vi "Lector_Ingen.vi"() -> ()   [LabVIEW 2017, in "Lib_Maestro_Ingen.lvlib"]
uses:
  Lib_Maestro_Ingen.lvlib
panel:
  in  "000001":bool
  in  "400001":u16
  in  "Tab Control 3":enum32{"Registro", "Control de variables"}(tab)=enum."Control de variables"
  in  "Tab Control":T1(tab)=enum."Registro de Frecuencia"
  out "Voltaje Fase 3":dbl(graph)=119.45
  out "Voltaje Fase 2":dbl(graph)=135.24
  out "Voltaje Fase 1":dbl(graph)=134.03
  out "Voltaje Promedio":dbl(graph)=233.23
  out "Corriente Promedio":dbl(graph)=53.75
  out "Corriente Fase 1":dbl(graph)=60.84
  out "Corriente Fase 2":dbl(graph)=61.24
  out "Corriente Fase 3":dbl(graph)=39.16
  out "Potencia Fase 3":dbl(graph)=76.8
  out "Potencia Fase 2":dbl(graph)=84.51
  out "Potencia Fase 1":dbl(graph)=83.64
  out "Potencia Promedio":dbl(graph)=81.65
  out "Factor de Potencia Fase 3":dbl(graph)=90.57
  out "Factor de Potencia Fase 2":dbl(graph)=90.84
  out "Factor de Potencia Fase 1":dbl(graph)=90.36
  out "Factor de Potencia Promedio":dbl(graph)=90.59
  out "Frecuencia":dbl(graph)=60.18
  in  "Tab Control 2":T2(tab)
  in  "CONTROL TEMPERATURA":cluster{"SET POINT":dbl, "INC T":dbl}={"SET POINT"=50.0, "INC T"=1.0}
  out "TEMPERATURA ACTUAL":dbl(slide)=31.0 scale=0.0..100.0
  out "Tempratura":cluster{"Dato":dbl, "SET POINT":dbl}(graph)
  out "Presion":cluster{"Dato":dbl, "SET POINT":dbl}(graph)
  in  "CONTROL DE PRESIÓN":cluster{"SET POINT":dbl, "INC P":dbl}={"SET POINT"=50.0, "INC P"=1.0}
  out "PRESIÓN ACTUAL":dbl(knob)=50.0 scale=0.0..200.0
  out "Humedad":cluster{"Dato":dbl, "SET POINT":dbl}(graph)
  in  "CONTROL DE HUMEDAD":cluster{"SET POINT":dbl, "INC %":dbl}={"SET POINT"=50.0, "INC %"=1.0}
  out "HUMEDAD ACTUAL":dbl(knob)=50.0 scale=0.0..100.0
  out "Volumen":cluster{"Dato":dbl, "SET POINT":dbl}(graph)
  in  "CONTROL DE LLENADO":cluster{"SET POINT":dbl, "INC  L":dbl}={"SET POINT"=25.0, "INC  L"=1.0}
  out "VOLUMEN ACTUAL":dbl(slide)=25.0 scale=0.0..100.0
  in  "Stop":bool
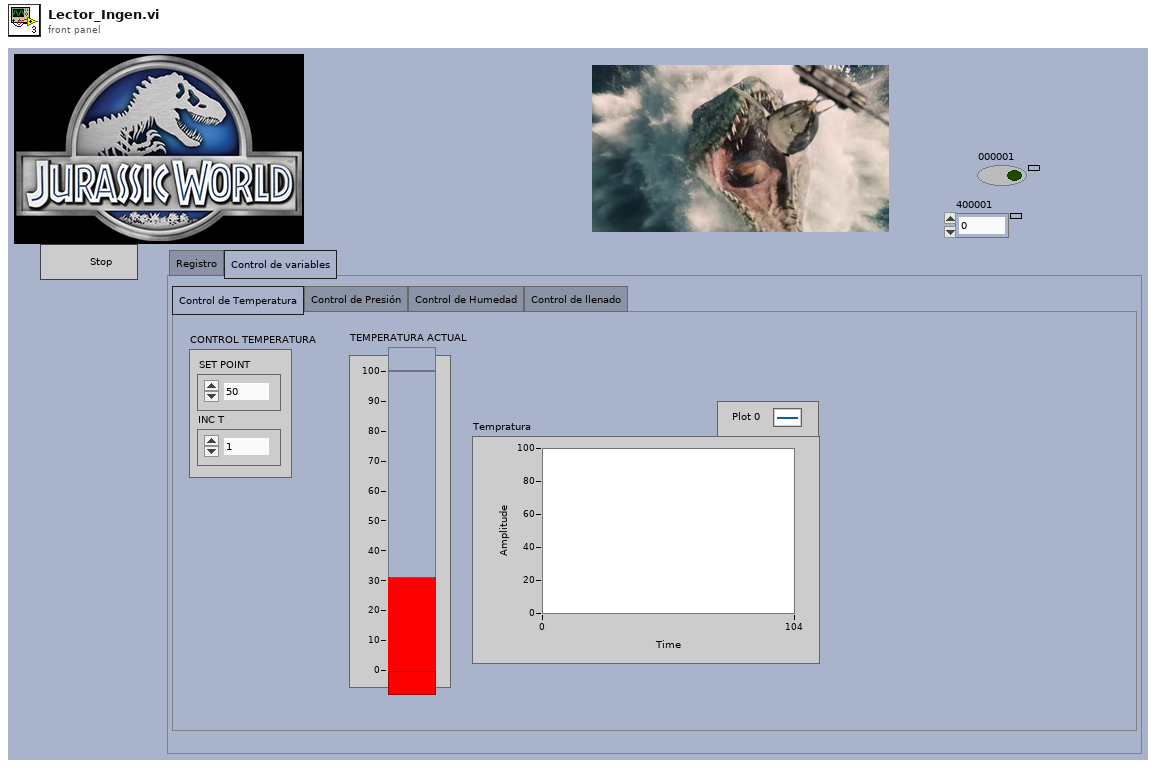
[diagram p1: front panel]
types:
  T1 = enum32{"Registro de Tensión", "Registro de Corriente", "Registro de Potencia", "Registro de Factor de Potencia", "Registro de Frecuencia"}
  T2 = enum32{"Control de Temperatura", "Control de Presión", "Control de Humedad", "Control de llenado"}
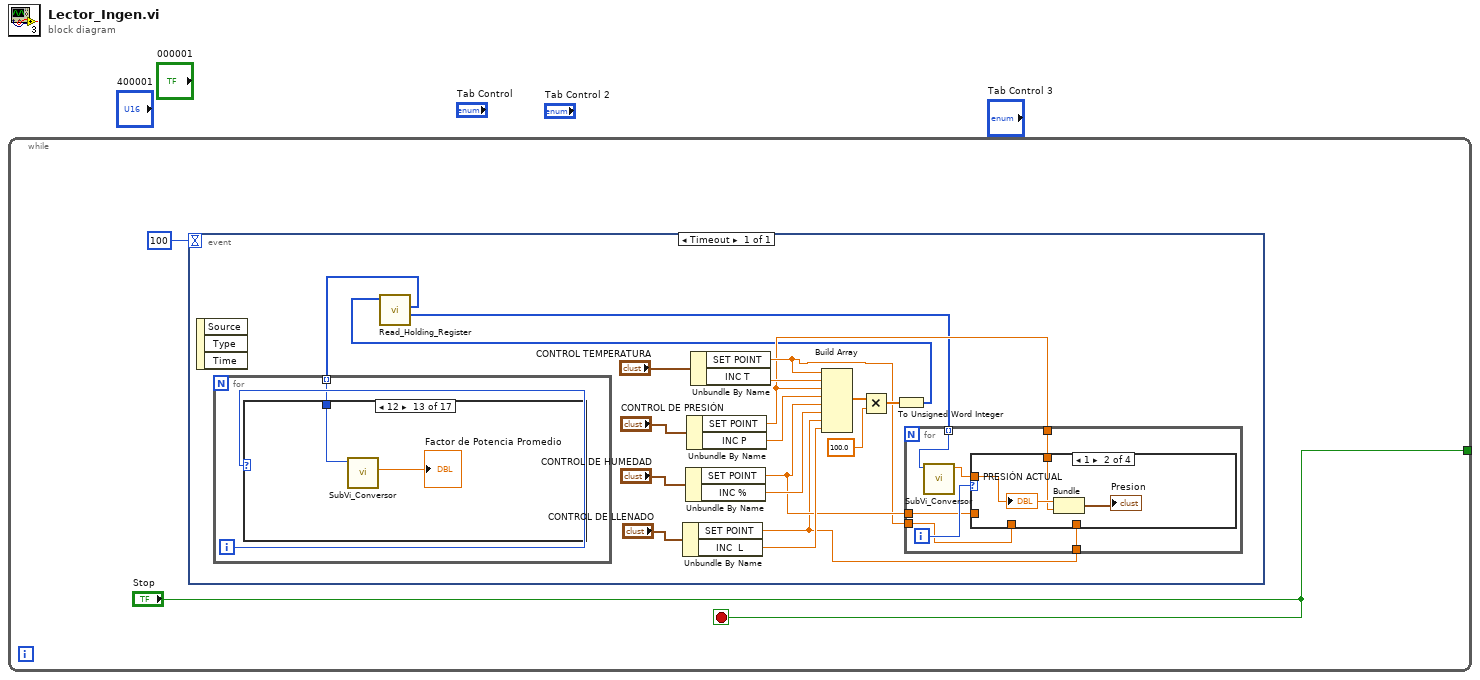
[diagram p0: block diagram]
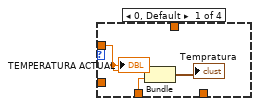
[diagram p2: hidden frame]
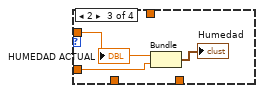
[diagram p3: hidden frame]
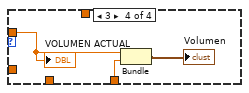
[diagram p4: hidden frame]
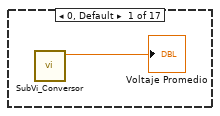
[diagram p5: hidden frame]
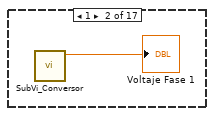
[diagram p6: hidden frame]
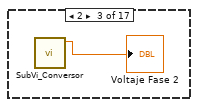
[diagram p7: hidden frame]
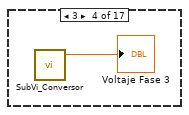
[diagram p8: hidden frame]
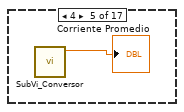
[diagram p9: hidden frame]
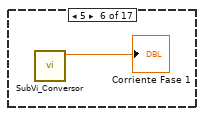
[diagram p10: hidden frame]
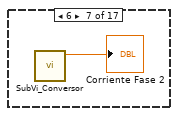
[diagram p11: hidden frame]
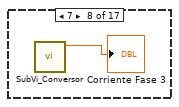
[diagram p12: hidden frame]
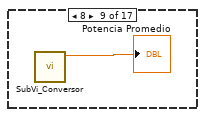
[diagram p13: hidden frame]
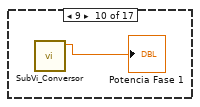
[diagram p14: hidden frame]
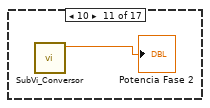
[diagram p15: hidden frame]
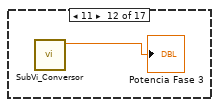
[diagram p16: hidden frame]
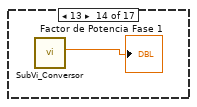
[diagram p17: hidden frame]
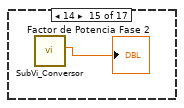
[diagram p18: hidden frame]
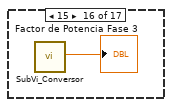
[diagram p19: hidden frame]
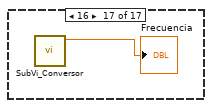
[diagram p20: hidden frame]
diagram:
  n1 = while {
    tunnel: ["Stop"] -> _
    stop <- "Stop" stop-if-true
    n2 = event shown="[0] Timeout" {
      selector: _ -> [_]
      dyn-events: _ -> [_]
      timeout: 100 -> [_]
      event Timeout {
        n3 = event-data() -> ()  [unwired: 1 in, 3 out]
        n4 = Unbundle By Name("CONTROL DE LLENADO") -> ("SET POINT"=w8:dbl, "INC  L"=w13:dbl)
        n5 = Unbundle By Name("CONTROL DE HUMEDAD") -> ("SET POINT"=w9:dbl, "INC %"=w14:dbl)
        n6 = Unbundle By Name("CONTROL DE PRESIÓN") -> ("SET POINT"=w6:dbl, "INC P"=w15:dbl)
        n7 = Unbundle By Name("CONTROL TEMPERATURA") -> ("SET POINT"=w7:dbl, "INC T"=w16:dbl)
        n8 = Build Array(w7, w16, w6, w15, w9, w14, w8, w13) -> (w12:dbl[])
        n9 = Multiply(x=w12, y=100.0) -> (x*y=w10:dbl[])
        n10 = To Unsigned Word Integer(number=w10) -> (unsigned 16bit integer=w5:u16[])
        n11 = call "Read_Holding_Register.vi"("Escritura_Variables"=w5) -> ("Registros_B"=w3:u16[], "Registros_A"=w4:u16[])  [unwired: 7 in, 1 out]
        n12 = for {
          tunnel: w4 -> [w40] mode=indexing
          i -> [w41]
          n13 = case shown="12" w41 {
            tunnel: w40 -> [_ _ _ _ _ _ _ _ _ _ _ _ w54 _ _ _ _]
            frame 0, Default {
              n14 = call "SubVi_Conversor.vi"() -> ("Dato"=→"Voltaje Promedio":dbl)  [unwired: 10 in, 1 out]
            }
            frame 1 {
              n15 = call "SubVi_Conversor.vi"() -> ("Dato"=→"Voltaje Fase 1":dbl)  [unwired: 10 in, 1 out]
            }
            frame 2 {
              n16 = call "SubVi_Conversor.vi"() -> ("Dato"=→"Voltaje Fase 2":dbl)  [unwired: 10 in, 1 out]
            }
            frame 3 {
              n17 = call "SubVi_Conversor.vi"() -> ("Dato"=→"Voltaje Fase 3":dbl)  [unwired: 10 in, 1 out]
            }
            frame 4 {
              n18 = call "SubVi_Conversor.vi"() -> ("Dato"=→"Corriente Promedio":dbl)  [unwired: 10 in, 1 out]
            }
            frame 5 {
              n19 = call "SubVi_Conversor.vi"() -> ("Dato"=→"Corriente Fase 1":dbl)  [unwired: 10 in, 1 out]
            }
            frame 6 {
              n20 = call "SubVi_Conversor.vi"() -> ("Dato"=→"Corriente Fase 2":dbl)  [unwired: 10 in, 1 out]
            }
            frame 7 {
              n21 = call "SubVi_Conversor.vi"() -> ("Dato"=→"Corriente Fase 3":dbl)  [unwired: 10 in, 1 out]
            }
            frame 8 {
              n22 = call "SubVi_Conversor.vi"() -> ("Dato"=→"Potencia Promedio":dbl)  [unwired: 10 in, 1 out]
            }
            frame 9 {
              n23 = call "SubVi_Conversor.vi"() -> ("Dato"=→"Potencia Fase 1":dbl)  [unwired: 10 in, 1 out]
            }
            frame 10 {
              n24 = call "SubVi_Conversor.vi"() -> ("Dato"=→"Potencia Fase 2":dbl)  [unwired: 10 in, 1 out]
            }
            frame 11 {
              n25 = call "SubVi_Conversor.vi"() -> ("Dato"=→"Potencia Fase 3":dbl)  [unwired: 10 in, 1 out]
            }
            frame 12 {
              n26 = call "SubVi_Conversor.vi"("Entrada_U16"=w54) -> ("Factor_de_potencia"=→"Factor de Potencia Promedio":dbl)  [unwired: 9 in, 1 out]
            }
            frame 13 {
              n27 = call "SubVi_Conversor.vi"() -> ("Factor_de_potencia"=→"Factor de Potencia Fase 1":dbl)  [unwired: 10 in, 1 out]
            }
            frame 14 {
              n28 = call "SubVi_Conversor.vi"() -> ("Factor_de_potencia"=→"Factor de Potencia Fase 2":dbl)  [unwired: 10 in, 1 out]
            }
            frame 15 {
              n29 = call "SubVi_Conversor.vi"() -> ("Factor_de_potencia"=→"Factor de Potencia Fase 3":dbl)  [unwired: 10 in, 1 out]
            }
            frame 16 {
              n30 = call "SubVi_Conversor.vi"() -> ("Dato"=→"Frecuencia":dbl)  [unwired: 10 in, 1 out]
            }
          }
        }
        n31 = for {
          tunnel: w9 -> [w25]
          tunnel: w8 -> [w24]
          tunnel: w7 -> [w23]
          tunnel: w6 -> [w22]
          tunnel: w3 -> [w21] mode=indexing
          i -> [w27]
          n32 = call "SubVi_Conversor.vi"("Entrada_U16"=w21) -> ("Dato"=w26:dbl)  [unwired: 9 in, 1 out]
          n33 = case shown="1" w27 {
            tunnel: w26 -> [w29 w32 w36 w38]
            tunnel: w25 -> [_ _ w34 _]
            tunnel: w24 -> [_ _ _ w37]
            tunnel: w23 -> [w28 _ _ _]
            tunnel: w22 -> [_ w31 _ _]
            frame 0, Default {
              n34 = Bundle("Dato"=w29, "SET POINT"=w28) -> (→"Tempratura":cluster{"Dato":dbl, "SET POINT":dbl})  [unwired: 1 in]
              "TEMPERATURA ACTUAL" <- w29
            }
            frame 1 {
              n35 = Bundle("Dato"=w32, "SET POINT"=w31) -> (→"Presion":cluster{"Dato":dbl, "SET POINT":dbl})  [unwired: 1 in]
              "PRESIÓN ACTUAL" <- w32
            }
            frame 2 {
              n36 = Bundle("Dato"=w36, "SET POINT"=w34) -> (→"Humedad":cluster{"Dato":dbl, "SET POINT":dbl})  [unwired: 1 in]
              "HUMEDAD ACTUAL" <- w36
            }
            frame 3 {
              n37 = Bundle("Dato"=w38, "SET POINT"=w37) -> (→"Volumen":cluster{"Dato":dbl, "SET POINT":dbl})  [unwired: 1 in]
              "VOLUMEN ACTUAL" <- w38
            }
          }
        }
      }
    }
  }
